vi "RtdeWriteInputs.vi"(8 "Data":T1, 10 "Rtde":refnum<k24>, 11 "error in":errorcluster) -> (3 "error out":errorcluster)   [LabVIEW 2022 SP3, in "UnderAutomation.UniversalRobots.lvlib"]
uses:
  UnderAutomation.UniversalRobots.lvlib
  C:/Users/fg/Documents/UniversalRobots.vi/LabVIEW_2023/UnderAutomation.UniversalRobots/lib/UnderAutomation.UniversalRobots.dll
  LabVIEW_2023/UnderAutomation.UniversalRobots/lib/UnderAutomation.UniversalRobots.dll
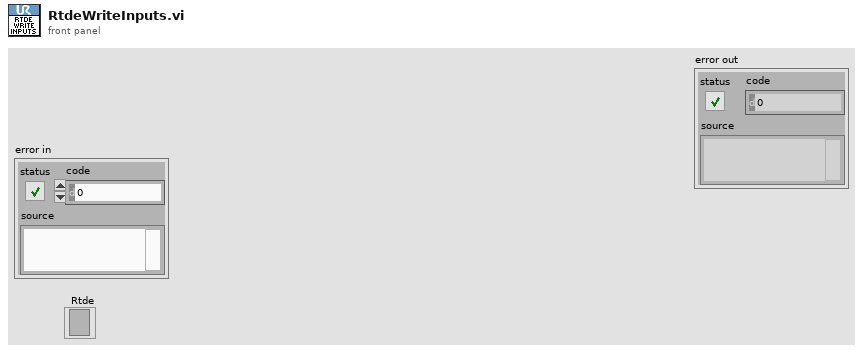
[diagram p1: front panel]
types:
  T1 = cluster{"ConfigurableDigitalOutput":u8, "ConfigurableDigitalOutputMask":u8, "ExternalForceTorque":cluster{"X":dbl, "Y":dbl, "Z":dbl, "Rx":dbl, "Ry":dbl, "Rz":dbl}, "InputBitRegisters":cluster{"X64":bool, "X65":bool, "X66":bool, "X67":bool, "X68":bool, "X69":bool, "X70":bool, "X71":bool, "X72":bool, "X73":bool, "X74":bool, "X75":bool, "X76":bool, "X77":bool, "X78":bool, "X79":bool, "X80":bool, "X81":bool, "X82":bool, "X83":bool, "X84":bool, "X85":bool, "X86":bool, "X87":bool, "X88":bool, "X89":bool, "X90":bool, "X91":bool, "X92":bool, "X93":bool, "X94":bool, "X95":bool, "X96":bool, "X97":bool, "X98":bool, "X99":bool, "X100":bool, "X101":bool, "X102":bool, "X103":bool, "X104":bool, "X105":bool, "X106":bool, "X107":bool, "X108":bool, "X109":bool, "X110":bool, "X111":bool, "X112":bool, "X113":bool, "X114":bool, "X115":bool, "X116":bool, "X117":bool, "X118":bool, "X119":bool, "X120":bool, "X121":bool, "X122":bool, "X123":bool, "X124":bool, "X125":bool, "X126":bool, "X127":bool}, "InputBtRegisters0To31":u32, "InputBtRegisters32To63":u32, "InputDoubleRegisters":cluster{"X0":dbl, "X1":dbl, "X2":dbl, "X3":dbl, "X4":dbl, "X5":dbl, "X6":dbl, "X7":dbl, "X8":dbl, "X9":dbl, "X10":dbl, "X11":dbl, "X12":dbl, "X13":dbl, "X14":dbl, "X15":dbl, "X16":dbl, "X17":dbl, "X18":dbl, "X19":dbl, "X20":dbl, "X21":dbl, "X22":dbl, "X23":dbl, "X24":dbl, "X25":dbl, "X26":dbl, "X27":dbl, "X28":dbl, "X29":dbl, "X30":dbl, "X31":dbl, "X32":dbl, "X33":dbl, "X34":dbl, "X35":dbl, "X36":dbl, "X37":dbl, "X38":dbl, "X39":dbl, "X40":dbl, "X41":dbl, "X42":dbl, "X43":dbl, "X44":dbl, "X45":dbl, "X46":dbl, "X47":dbl}, "InputIntRegisters":cluster{"X0":i32, "X1":i32, "X2":i32, "X3":i32, "X4":i32, "X5":i32, "X6":i32, "X7":i32, "X8":i32, "X9":i32, "X10":i32, "X11":i32, "X12":i32, "X13":i32, "X14":i32, "X15":i32, "X16":i32, "X17":i32, "X18":i32, "X19":i32, "X20":i32, "X21":i32, "X22":i32, "X23":i32, "X24":i32, "X25":i32, "X26":i32, "X27":i32, "X28":i32, "X29":i32, "X30":i32, "X31":i32, "X32":i32, "X33":i32, "X34":i32, "X35":i32, "X36":i32, "X37":i32, "X38":i32, "X39":i32, "X40":i32, "X41":i32, "X42":i32, "X43":i32, "X44":i32, "X45":i32, "X46":i32, "X47":i32}, "SpeedSliderFraction":dbl, "SpeedSliderMask":u32, "StandardAnalogOutput0":dbl, "StandardAnalogOutput1":dbl, "StandardAnalogOutputMask":u8, "StandardAnalogOutputType":u8, "StandardDigitalOutput":u8, "StandardDigitalOutputMask":u8}
  T2 = cluster{"X":dbl, "Y":dbl, "Z":dbl, "Rx":dbl, "Ry":dbl, "Rz":dbl}
  T3 = cluster{"X64":bool, "X65":bool, "X66":bool, "X67":bool, "X68":bool, "X69":bool, "X70":bool, "X71":bool, "X72":bool, "X73":bool, "X74":bool, "X75":bool, "X76":bool, "X77":bool, "X78":bool, "X79":bool, "X80":bool, "X81":bool, "X82":bool, "X83":bool, "X84":bool, "X85":bool, "X86":bool, "X87":bool, "X88":bool, "X89":bool, "X90":bool, "X91":bool, "X92":bool, "X93":bool, "X94":bool, "X95":bool, "X96":bool, "X97":bool, "X98":bool, "X99":bool, "X100":bool, "X101":bool, "X102":bool, "X103":bool, "X104":bool, "X105":bool, "X106":bool, "X107":bool, "X108":bool, "X109":bool, "X110":bool, "X111":bool, "X112":bool, "X113":bool, "X114":bool, "X115":bool, "X116":bool, "X117":bool, "X118":bool, "X119":bool, "X120":bool, "X121":bool, "X122":bool, "X123":bool, "X124":bool, "X125":bool, "X126":bool, "X127":bool}
  T4 = cluster{"X0":dbl, "X1":dbl, "X2":dbl, "X3":dbl, "X4":dbl, "X5":dbl, "X6":dbl, "X7":dbl, "X8":dbl, "X9":dbl, "X10":dbl, "X11":dbl, "X12":dbl, "X13":dbl, "X14":dbl, "X15":dbl, "X16":dbl, "X17":dbl, "X18":dbl, "X19":dbl, "X20":dbl, "X21":dbl, "X22":dbl, "X23":dbl, "X24":dbl, "X25":dbl, "X26":dbl, "X27":dbl, "X28":dbl, "X29":dbl, "X30":dbl, "X31":dbl, "X32":dbl, "X33":dbl, "X34":dbl, "X35":dbl, "X36":dbl, "X37":dbl, "X38":dbl, "X39":dbl, "X40":dbl, "X41":dbl, "X42":dbl, "X43":dbl, "X44":dbl, "X45":dbl, "X46":dbl, "X47":dbl}
  T5 = cluster{"X0":i32, "X1":i32, "X2":i32, "X3":i32, "X4":i32, "X5":i32, "X6":i32, "X7":i32, "X8":i32, "X9":i32, "X10":i32, "X11":i32, "X12":i32, "X13":i32, "X14":i32, "X15":i32, "X16":i32, "X17":i32, "X18":i32, "X19":i32, "X20":i32, "X21":i32, "X22":i32, "X23":i32, "X24":i32, "X25":i32, "X26":i32, "X27":i32, "X28":i32, "X29":i32, "X30":i32, "X31":i32, "X32":i32, "X33":i32, "X34":i32, "X35":i32, "X36":i32, "X37":i32, "X38":i32, "X39":i32, "X40":i32, "X41":i32, "X42":i32, "X43":i32, "X44":i32, "X45":i32, "X46":i32, "X47":i32}
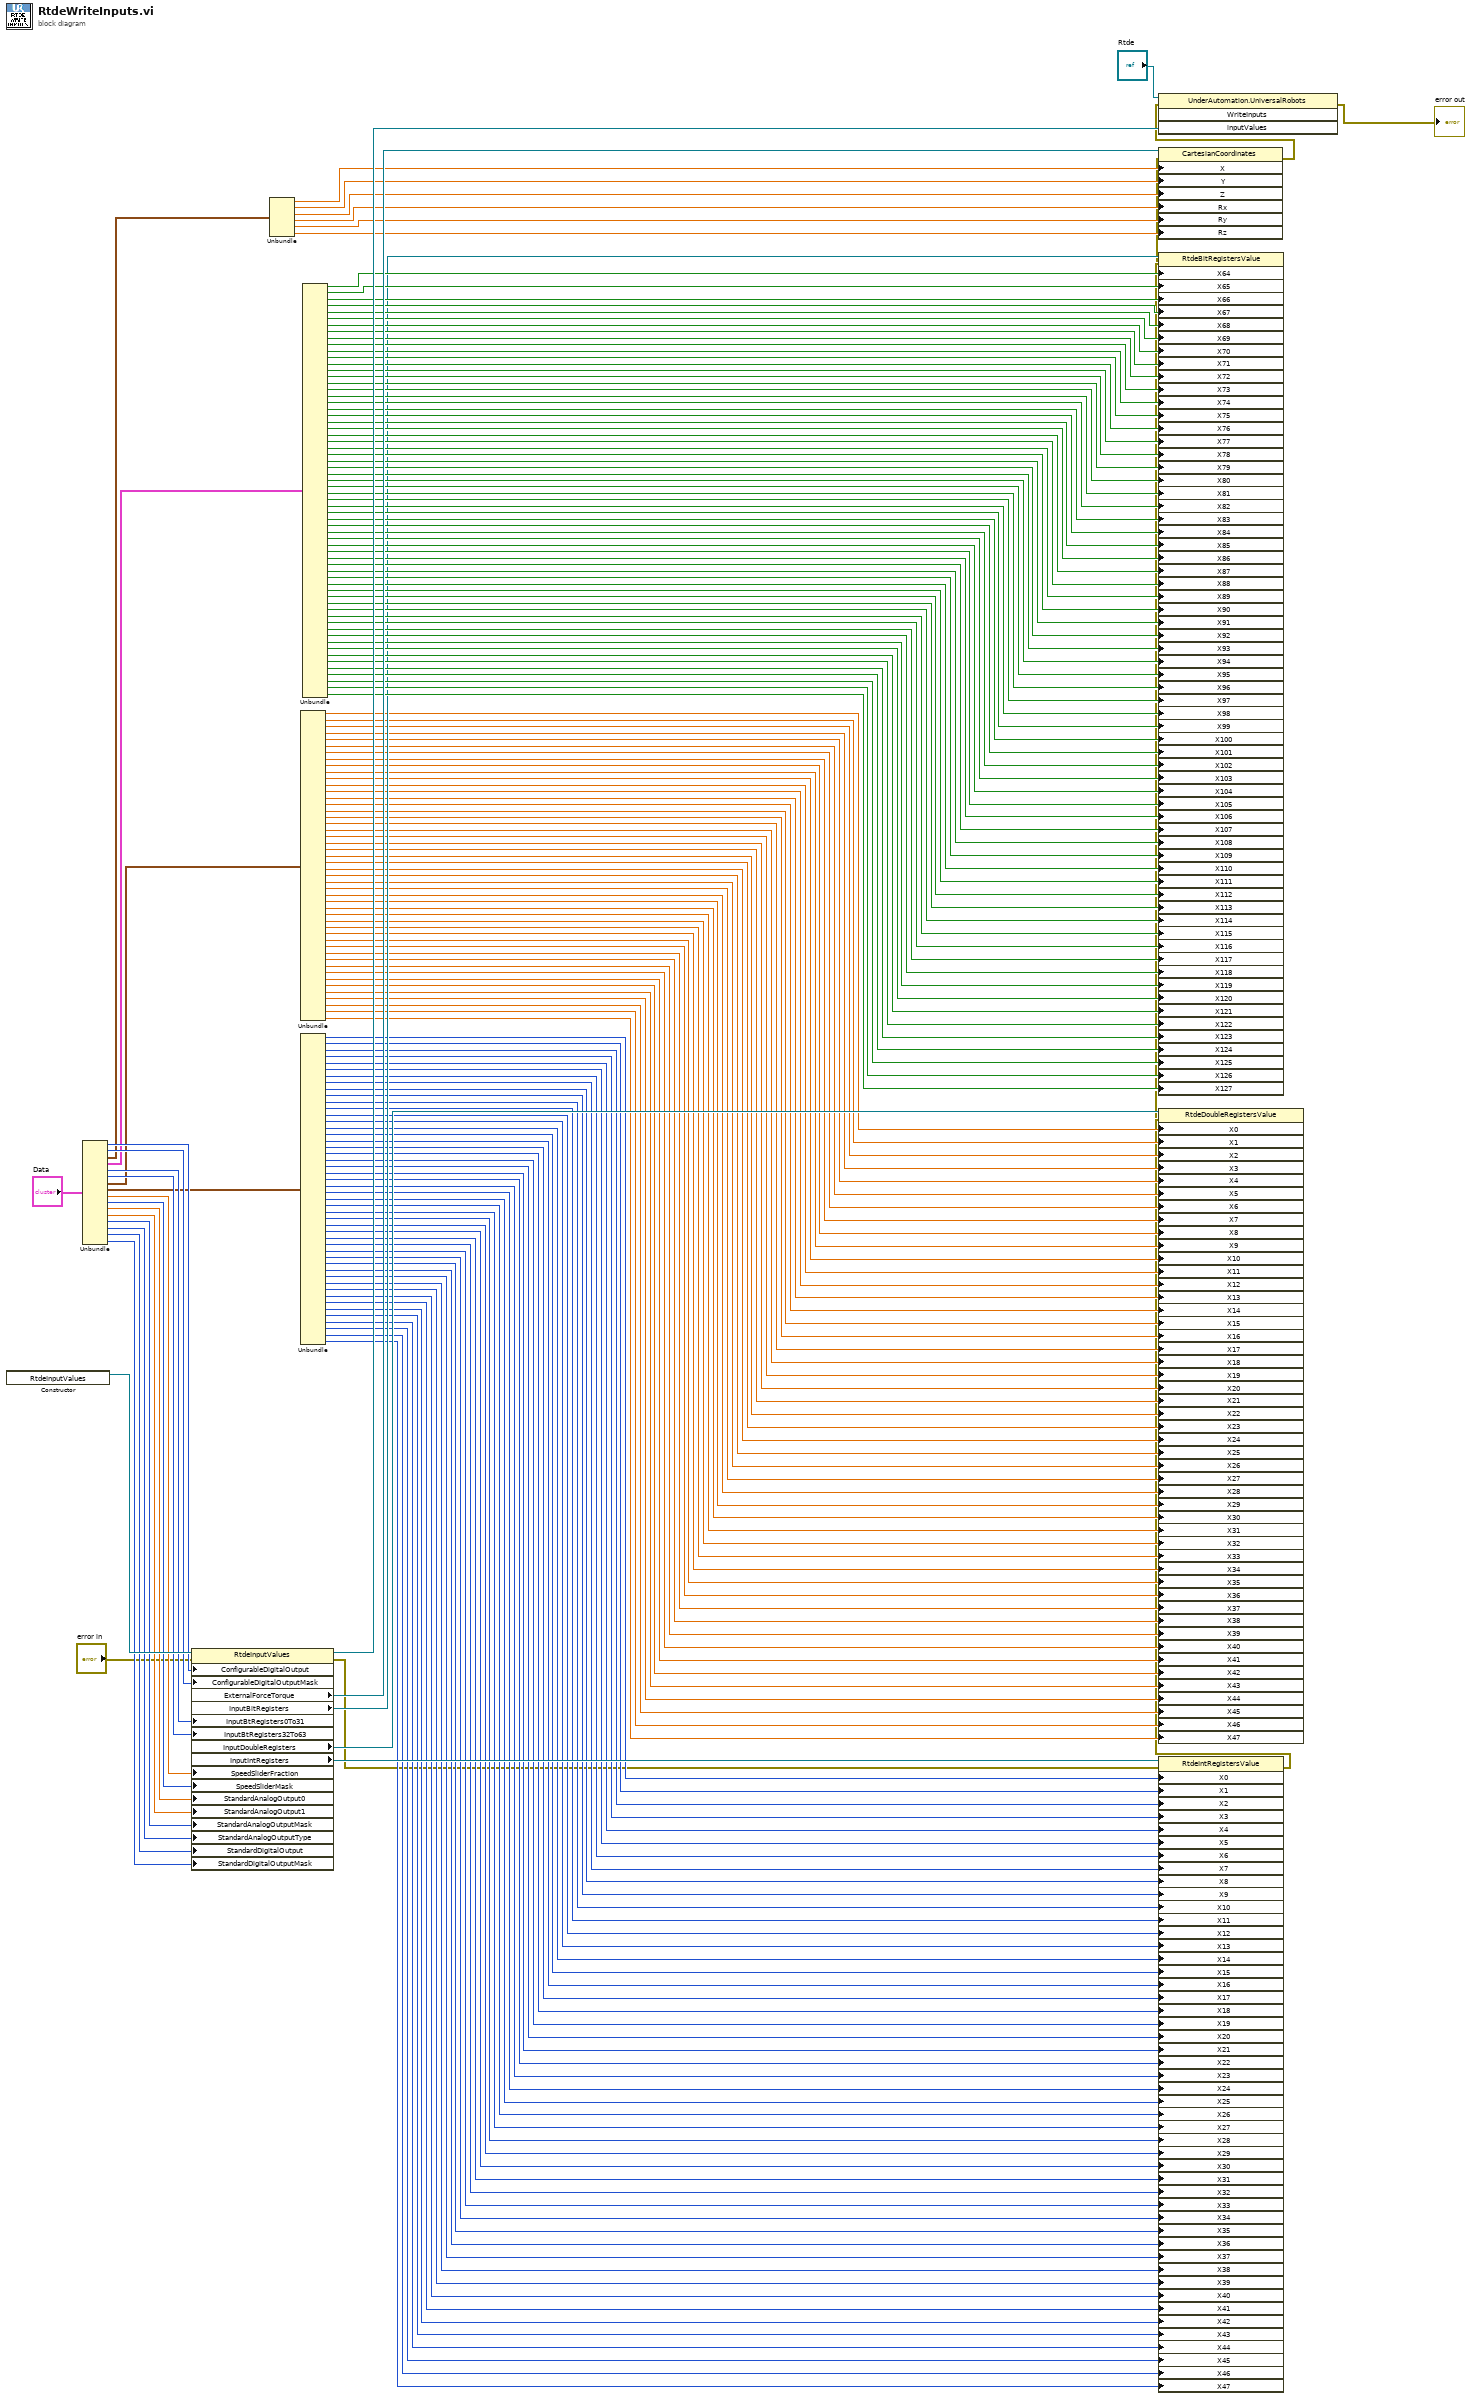
[diagram p0: block diagram]
diagram:
  n1 = constructor class="RtdeInputValues"() -> (reference out=w196:refnum<k24>)  [unwired: 3 in, 2 out]
  n2 = Unbundle("Data") -> ("ConfigurableDigitalOutput"=w193:u8, "ConfigurableDigitalOutputMask"=w192:u8, "ExternalForceTorque"=w181:T2, "InputBitRegisters"=w173:T3, "InputBtRegisters0To31"=w191:u32, "InputBtRegisters32To63"=w190:u32, "InputDoubleRegisters"=w108:T4, "InputIntRegisters"=w56:T5, "SpeedSliderFraction"=w189:dbl, "SpeedSliderMask"=w188:u32, "StandardAnalogOutput0"=w187:dbl, "StandardAnalogOutput1"=w186:dbl, "StandardAnalogOutputMask"=w185:u8, "StandardAnalogOutputType"=w184:u8, "StandardDigitalOutput"=w183:u8, "StandardDigitalOutputMask"=w182:u8)
  n3 = property class="RtdeInputValues"(reference=w196, error in="error in", "ConfigurableDigitalOutput"=w193, "ConfigurableDigitalOutputMask"=w192, "InputBtRegisters0To31"=w191, "InputBtRegisters32To63"=w190, "SpeedSliderFraction"=w189, "SpeedSliderMask"=w188, "StandardAnalogOutput0"=w187, "StandardAnalogOutput1"=w186, "StandardAnalogOutputMask"=w185, "StandardAnalogOutputType"=w184, "StandardDigitalOutput"=w183, "StandardDigitalOutputMask"=w182) -> (reference out=w195:refnum<k24>, error out=w6:errorcluster, "ExternalForceTorque"=w180:refnum<k24>, "InputBitRegisters"=w107:refnum<k24>, "InputDoubleRegisters"=w106:refnum<k24>, "InputIntRegisters"=w57:refnum<k24>)
  n4 = Unbundle(w181) -> ("X"=w179:dbl, "Y"=w178:dbl, "Z"=w176:dbl, "Rx"=w177:dbl, "Ry"=w175:dbl, "Rz"=w174:dbl)
  n5 = Unbundle(w108) -> ("X0"=w105:dbl, "X1"=w104:dbl, "X2"=w103:dbl, "X3"=w102:dbl, "X4"=w101:dbl, "X5"=w100:dbl, "X6"=w99:dbl, "X7"=w98:dbl, "X8"=w97:dbl, "X9"=w96:dbl, "X10"=w95:dbl, "X11"=w94:dbl, "X12"=w93:dbl, "X13"=w92:dbl, "X14"=w89:dbl, "X15"=w91:dbl, "X16"=w90:dbl, "X17"=w88:dbl, "X18"=w87:dbl, "X19"=w86:dbl, "X20"=w85:dbl, "X21"=w84:dbl, "X22"=w83:dbl, "X23"=w82:dbl, "X24"=w81:dbl, "X25"=w80:dbl, "X26"=w79:dbl, "X27"=w78:dbl, "X28"=w77:dbl, "X29"=w76:dbl, "X30"=w75:dbl, "X31"=w74:dbl, "X32"=w73:dbl, "X33"=w72:dbl, "X34"=w71:dbl, "X35"=w69:dbl, "X36"=w70:dbl, "X37"=w68:dbl, "X38"=w67:dbl, "X39"=w66:dbl, "X40"=w65:dbl, "X41"=w64:dbl, "X42"=w63:dbl, "X43"=w62:dbl, "X44"=w61:dbl, "X45"=w60:dbl, "X46"=w59:dbl, "X47"=w58:dbl)
  n6 = Unbundle(w56) -> ("X0"=w55:i32, "X1"=w54:i32, "X2"=w53:i32, "X3"=w52:i32, "X4"=w51:i32, "X5"=w50:i32, "X6"=w49:i32, "X7"=w48:i32, "X8"=w47:i32, "X9"=w46:i32, "X10"=w45:i32, "X11"=w44:i32, "X12"=w43:i32, "X13"=w42:i32, "X14"=w41:i32, "X15"=w40:i32, "X16"=w39:i32, "X17"=w38:i32, "X18"=w37:i32, "X19"=w36:i32, "X20"=w35:i32, "X21"=w34:i32, "X22"=w33:i32, "X23"=w32:i32, "X24"=w31:i32, "X25"=w30:i32, "X26"=w29:i32, "X27"=w28:i32, "X28"=w27:i32, "X29"=w26:i32, "X30"=w25:i32, "X31"=w24:i32, "X32"=w23:i32, "X33"=w22:i32, "X34"=w21:i32, "X35"=w20:i32, "X36"=w19:i32, "X37"=w18:i32, "X38"=w16:i32, "X39"=w17:i32, "X40"=w15:i32, "X41"=w14:i32, "X42"=w13:i32, "X43"=w12:i32, "X44"=w11:i32, "X45"=w10:i32, "X46"=w9:i32, "X47"=w8:i32)
  n7 = Unbundle(w173) -> ("X64"=w172:bool, "X65"=w171:bool, "X66"=w170:bool, "X67"=w169:bool, "X68"=w168:bool, "X69"=w167:bool, "X70"=w166:bool, "X71"=w165:bool, "X72"=w164:bool, "X73"=w163:bool, "X74"=w162:bool, "X75"=w161:bool, "X76"=w160:bool, "X77"=w159:bool, "X78"=w158:bool, "X79"=w157:bool, "X80"=w156:bool, "X81"=w155:bool, "X82"=w154:bool, "X83"=w153:bool, "X84"=w152:bool, "X85"=w151:bool, "X86"=w150:bool, "X87"=w149:bool, "X88"=w148:bool, "X89"=w147:bool, "X90"=w146:bool, "X91"=w145:bool, "X92"=w144:bool, "X93"=w143:bool, "X94"=w142:bool, "X95"=w141:bool, "X96"=w140:bool, "X97"=w139:bool, "X98"=w138:bool, "X99"=w137:bool, "X100"=w136:bool, "X101"=w135:bool, "X102"=w134:bool, "X103"=w133:bool, "X104"=w132:bool, "X105"=w131:bool, "X106"=w130:bool, "X107"=w129:bool, "X108"=w128:bool, "X109"=w127:bool, "X110"=w126:bool, "X111"=w125:bool, "X112"=w124:bool, "X113"=w123:bool, "X114"=w122:bool, "X115"=w121:bool, "X116"=w120:bool, "X117"=w119:bool, "X118"=w117:bool, "X119"=w118:bool, "X120"=w116:bool, "X121"=w115:bool, "X122"=w114:bool, "X123"=w113:bool, "X124"=w112:bool, "X125"=w111:bool, "X126"=w110:bool, "X127"=w109:bool)
  n8 = property class="RtdeIntRegistersValue"(reference=w57, error in=w6, "X0"=w55, "X1"=w54, "X2"=w53, "X3"=w52, "X4"=w51, "X5"=w50, "X6"=w49, "X7"=w48, "X8"=w47, "X9"=w46, "X10"=w45, "X11"=w44, "X12"=w43, "X13"=w42, "X14"=w41, "X15"=w40, "X16"=w39, "X17"=w38, "X18"=w37, "X19"=w36, "X20"=w35, "X21"=w34, "X22"=w33, "X23"=w32, "X24"=w31, "X25"=w30, "X26"=w29, "X27"=w28, "X28"=w27, "X29"=w26, "X30"=w25, "X31"=w24, "X32"=w23, "X33"=w22, "X34"=w21, "X35"=w20, "X36"=w19, "X37"=w18, "X38"=w16, "X39"=w17, "X40"=w15, "X41"=w14, "X42"=w13, "X43"=w12, "X44"=w11, "X45"=w10, "X46"=w9, "X47"=w8) -> (error out=w5:errorcluster)  [unwired: 1 out]
  n9 = property class="RtdeDoubleRegistersValue"(reference=w106, error in=w5, "X0"=w105, "X1"=w104, "X2"=w103, "X3"=w102, "X4"=w101, "X5"=w100, "X6"=w99, "X7"=w98, "X8"=w97, "X9"=w96, "X10"=w95, "X11"=w94, "X12"=w93, "X13"=w92, "X14"=w89, "X15"=w91, "X16"=w90, "X17"=w88, "X18"=w87, "X19"=w86, "X20"=w85, "X21"=w84, "X22"=w83, "X23"=w82, "X24"=w81, "X25"=w80, "X26"=w79, "X27"=w78, "X28"=w77, "X29"=w76, "X30"=w75, "X31"=w74, "X32"=w73, "X33"=w72, "X34"=w71, "X35"=w69, "X36"=w70, "X37"=w68, "X38"=w67, "X39"=w66, "X40"=w65, "X41"=w64, "X42"=w63, "X43"=w62, "X44"=w61, "X45"=w60, "X46"=w59, "X47"=w58) -> (error out=w4:errorcluster)  [unwired: 1 out]
  n10 = property class="RtdeBitRegistersValue"(reference=w107, error in=w4, "X64"=w172, "X65"=w171, "X66"=w170, "X67"=w169, "X68"=w168, "X69"=w167, "X70"=w166, "X71"=w165, "X72"=w164, "X73"=w163, "X74"=w162, "X75"=w161, "X76"=w160, "X77"=w159, "X78"=w158, "X79"=w157, "X80"=w156, "X81"=w155, "X82"=w154, "X83"=w153, "X84"=w152, "X85"=w151, "X86"=w150, "X87"=w149, "X88"=w148, "X89"=w147, "X90"=w146, "X91"=w145, "X92"=w144, "X93"=w143, "X94"=w142, "X95"=w141, "X96"=w140, "X97"=w139, "X98"=w138, "X99"=w137, "X100"=w136, "X101"=w135, "X102"=w134, "X103"=w133, "X104"=w132, "X105"=w131, "X106"=w130, "X107"=w129, "X108"=w128, "X109"=w127, "X110"=w126, "X111"=w125, "X112"=w124, "X113"=w123, "X114"=w122, "X115"=w121, "X116"=w120, "X117"=w119, "X118"=w117, "X119"=w118, "X120"=w116, "X121"=w115, "X122"=w114, "X123"=w113, "X124"=w112, "X125"=w111, "X126"=w110, "X127"=w109) -> (error out=w3:errorcluster)  [unwired: 1 out]
  n11 = property class="CartesianCoordinates"(reference=w180, error in=w3, "X"=w179, "Y"=w178, "Z"=w176, "Rx"=w177, "Ry"=w175, "Rz"=w174) -> (error out=w2:errorcluster)  [unwired: 1 out]
  n12 = invoke class="UnderAutomation.UniversalRobots" method="WriteInputs"(reference="Rtde", error in=w2, "inputValues"=w195) -> (error out=→"error out":errorcluster)  [unwired: 1 in, 3 out]
